vi "Reserve Device.vi"(8 "error in (no error)":errorcluster, 11 "SLSC Switch in":refnum<class "SLSC Switch.lvclass">) -> (0 "error out":errorcluster, 3 "SLSC Switch out":refnum<class "SLSC Switch.lvclass">)   [LabVIEW 2015, in "SLSC Switch.lvlib" / "SLSC Switch.lvclass"]
uses:
  SLSC Switch.lvclass
  SLSC Switch.lvclass/SLSC Switch.ctl
  <vilib>/National Instruments/SLSC Local or Remote Interface/SLSC Interface Class/SLSC Interface.lvclass
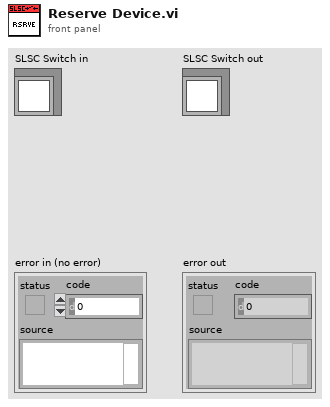
[diagram p1: front panel]
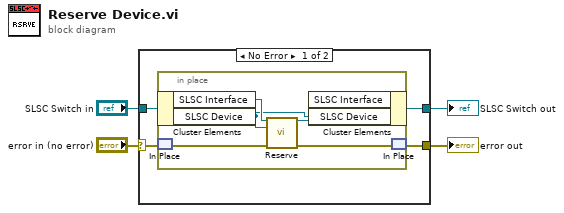
[diagram p0: block diagram]
diagram:
  n1 = case shown="No Error" "error in (no error)" {
    selector: "error in (no error)" -> [w7 w15]
    tunnel: [w6 w15] -> w3
    tunnel: [w5 w14] -> w1
    tunnel: "SLSC Switch in" -> [w8 w14]
    frame No Error {
      n2 = in-place {
        n3 = in-place-cluster #1(w8) -> ("SLSC Interface"=w13:refnum<class "SLSC Interface.lvclass">, "SLSC Device"=w9:refnum<k21>)
        n4 = in-place-match #2(w7) -> (w11:errorcluster)
        n5 = call-dynamic "Reserve.vi"("SLSC Interface in"=w13, "devices"=w9, "error in (no error)"=w11) -> ("SLSC Interface out"=w12:refnum<class "SLSC Interface.lvclass">, "error out"=w10:errorcluster)  [unwired: 11 in]
        n6 = in-place-cluster #1("SLSC Interface"=w12, "SLSC Device"=w9) -> (w5:refnum<class "SLSC Switch.lvclass">)
        n7 = in-place-match #2(w10) -> (w6:errorcluster)
      }
    }
    frame Error {
    }
  }
  "error out" <- w3
  "SLSC Switch out" <- w1
